vi "Update Motor Angle States.vi"(8 "error in (no error)":errorcluster, 10 "angles":dbl[](array[numeric]), 11 "motor communication in":refnum<class "NI_Robotics_Motor Communication.lvclass">[](array[class])) -> (0 "error out":errorcluster, 1 "failed?":bool[](array[boolean]), 3 "motor communication out":refnum<class "NI_Robotics_Motor Communication.lvclass">[](array[class]))   [LabVIEW 2017, in "NI_Robotics_Motor Communication.lvclass"]
doc: "Writes angle or angular velocity values of the motor or motors to the motor communication session. You must manually select the polymorphic instance to use."
uses:
  <vilib>/robotics/Actuation/Motor Communication/NI_Robotics_Motor Communication.lvclass
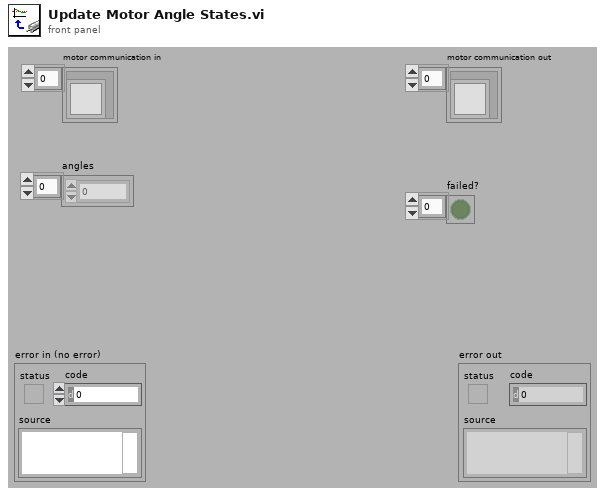
[diagram p1: front panel]
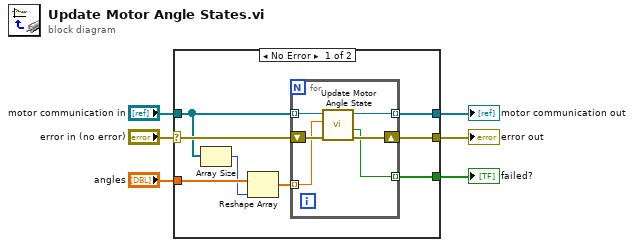
[diagram p0: block diagram]
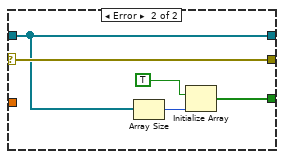
[diagram p2: hidden frame]
diagram:
  n1 = case shown="No Error" "error in (no error)" {
    selector: "error in (no error)" -> [w14 w25]
    tunnel: [w11 w25] -> w5
    tunnel: "motor communication in" -> [w10 w24]
    tunnel: "angles" -> [w9 _]
    tunnel: [w13 w21] -> w2
    tunnel: [w12 w24] -> w1
    frame No Error {
      n2 = Array Size(array=w10) -> (size(s)=w7:i32)
      n3 = Reshape Array(w9, w7) -> (w8:dbl[])
      n4 = for {
        tunnel: w10 -> [w20] mode=indexing
        tunnel: w8 -> [w18] mode=indexing
        shift-right: [w17] -> w11
        shift-left: w14 -> [w19]
        tunnel: [w16] -> w13 mode=indexing
        tunnel: [w15] -> w12 mode=indexing
        n5 = call <vilib>:"Update Motor Angle State.vi"("error in (no error)"=w19, "angle"=w18, "motor communication in"=w20) -> ("error out"=w17:errorcluster, "failed?"=w16:bool, "motor communication out"=w15:refnum<class "NI_Robotics_Motor Communication.lvclass">)  [unwired: 6 in]
      }
    }
    frame Error {
      n6 = Array Size(array=w24) -> (size(s)=w23:i32)
      n7 = Initialize Array(TRUE, w23) -> (w21:bool[])
    }
  }
  "error out" <- w5
  "motor communication out" <- w1
  "failed?" <- w2
